vi "Meas Result Generate TWM Digitizer Correction - Process Measurement.vi"(4 "Estimate non-linearity (False)":bool, 5 "digitizer type":T1=enum."HP3458A", 6 "use aperture correction (true)":bool=TRUE, 7 "table ref":refnum<vi>, 8 "error in":errorcluster, 9 "use time shift (true)":bool=TRUE, 10 "Mode":T3, 11 "meas":T4={"swp cfg"={"N"=0, "R"=0, "f list"=[], "smpl delay"=0.0, "set delay"=0.0, "set delay np"=0.0, "meas root"=path "", "meas name"="", "meas a-index"=FALSE, "rnd sweep"=FALSE, "mode"=enum."Frequency", "swp mode"=enum."Linear", "avg"=0, "subrec"=0, "multi-freq"=FALSE, "selfcal"=FALSE, "selfcal period [h]"=0.0}, "bridge"={"type"=enum."TWM client", "TWM"={"pipe name"="", "parameters"=[], "handle"=0, "fixed aper [s]"=0.0, "f-list [Hz]"=[], "discrete f-list"=FALSE, "unc mode"=enum."None", "unc mcc"=0, "unc first"=FALSE, "alg id"=enum."TWM-LowZ - Low Z measurement"}, "last f"=0.0, "bias comp"={"bias type"=enum."dummy", "VISA"="", "Enable"=FALSE, "channel qu"=[], "channel Uinit"=[]}, "sim mode"=enum."Generic RLC network", "channel idns"=[], "sim phases"=1}, "src"={"type"=enum."Tektronix AFG3101C", "afg"={"VISA"="", "const"=0.0, "gen DC"=FALSE, "ext ref"=FALSE}, "cDAQ dds"={"device"="", "channels"=[], "mclk source"="", "mclk [Hz]"=0.0, "fs [Hz]"=0.0, "block [s]"=0.0, "buf [s]"=0.0, "task"="", "cmd queue"=refnum, "proc ref"=refnum, "smpl clock out"="/cDAQ3/PFI0", "export smpl clock"=FALSE, "DC ofs [V]"=[], "timebase source"="", "timebase mode"=enum."Local", "dither"=enum."Disabled", "dither level"=0.0, "phase [rad]"=[]}, "gain [V/A]"=1.0, "F5xxx session"={"VISA"="", "mode"=enum."AC voltage", "Earth on"=FALSE, "Ext ref lock"=FALSE}}, "results"=refnum, "dvm"={"type"=enum."Disabled", "F5790"={"VISA"="", "Input"=enum."input 1", "Digital filter restart"=enum."medium", "hi resolution"=enum."off", "Digital filter mode"=enum."off", "ext guard"=FALSE}}, "thermo"={"type"=enum."COMET Tx5xx (ethernet)", "comment"="", "tag"="", "refresh"=5.0, "IP"="", "port"=502, "VISA"="", "last readout"=timestamp(0 s since 1904-01-01), "TCP ref"=refnum, "VISA sess"="", "idn"="", "press"=0.0, "RH"=0.0, "temp"=0.0, "pres cor"=[], "RH cor"=[], "temp cor"=[], "try left"=0, "failed"=FALSE, "RTD set"=[], "RTD inv"=[], "range"=0.0, "net mode"=enum."MODBUS", "try fail"=enum."Stop trying - return NaN", "timeout [s]"=0.0, "max retries"=0, "sim t [deg]"=0.0}} {"thermo"."RTD inv" format="%.1f"; "thermo"."RTD set" format="%.1f"; "thermo"."temp cor" format="%.1f"; "thermo"."RH cor" format="%.1f"; "thermo"."pres cor" format="%.1f"; "thermo"."refresh" min=0.1 max=1000.0 format="%.2f"; "src"."cDAQ dds"."channels" min=0 step=1; "bridge"."TWM"."f-list [Hz]" format="%#_6p"; "swp cfg"."f list"."bias" format="%#_3p"; "swp cfg"."f list"."level" format="%#_3p"; "swp cfg"."f list"."fs [Hz]" format="%#_5p"; "swp cfg"."f list"."time [s]" format="%#_3p"; "swp cfg"."f list"."f/fs" format="%#_3p"; "swp cfg"."f list"."periods" format="%#_3f"; "swp cfg"."f list"."f [Hz]" format="%#_5p"}) -> (0 "error out":errorcluster, 3 "correction data":T2)   [LabVIEW 2020]
doc: "Generates simple TWM digitizer correction from measured data."
uses:
  meas session.ctl
  Meas Sweep Config.ctl
  Meas Freq Info.ctl
  meas_swp_mode.ctl
  meas_sweep_flist_mode.ctl
  bridge/Bridge Session.ctl
  bridge/Bridge Type.ctl
  drivers/TWM client/TWM Session.ctl
  drivers/TWM client/TWM parameters.ctl
  drivers/TWM client/Meas Proc QWTB Uncertainty Mode.ctl
  bridge/Bridge Algorithm.ctl
  bridge/Bridge Bias Session.ctl
  bridge/Bridge Bias Type.ctl
  bridge/Bridge Sim Mode.ctl
  source/Source Session.ctl
  source/Source Type.ctl
  drivers/AFG3101C/AFG3101C Session.ctl
  drivers/cDAQ DDS/cDAQ DDS Session.ctl
  drivers/cDAQ DDS/cDAQ DDS Setup.ctl
  drivers/cDAQ DDS/cDAQ DDS Timebase Mode.ctl
  drivers/cDAQ DDS/cDAQ DDS Dither.ctl
  drivers/Fluke 5XXX/top_lev/F5xxx_session.ctl
  drivers/Fluke 5XXX/top_lev/F5xxx_output_mode.ctl
  results/Meas Results Ref.ctl
  results/Meas Results.ctl
  bridge/Bridge Frequency Readings Data.ctl
  drivers/TWM client/Meas Proc QWTB Spectrum Data.ctl
  drivers/TWM client/TWM Phase Info.ctl
  dvm/dvm session.ctl
  dvm/dvm type.ctl
  drivers/Fluke 5790A/top_level/F5790 session.ctl
  thermo/thermo.ctl
  thermo/thermo_types.ctl
  thermo/Thermometer Fail Action.ctl
  results/Meas Results Correction Structuring Mode.ctl
  Meas Results TWM Digitizer Correction Data.ctl
  Meas Results TWM Correction Digitizer Type.ctl
  results/Meas Results Sweep Data Uncertainty Mode.ctl
  results/Impedance Equivalent Circuit.ctl
panel:
  out "time shifts [s]":dbl[][](array[numeric]) format="%#_6p"
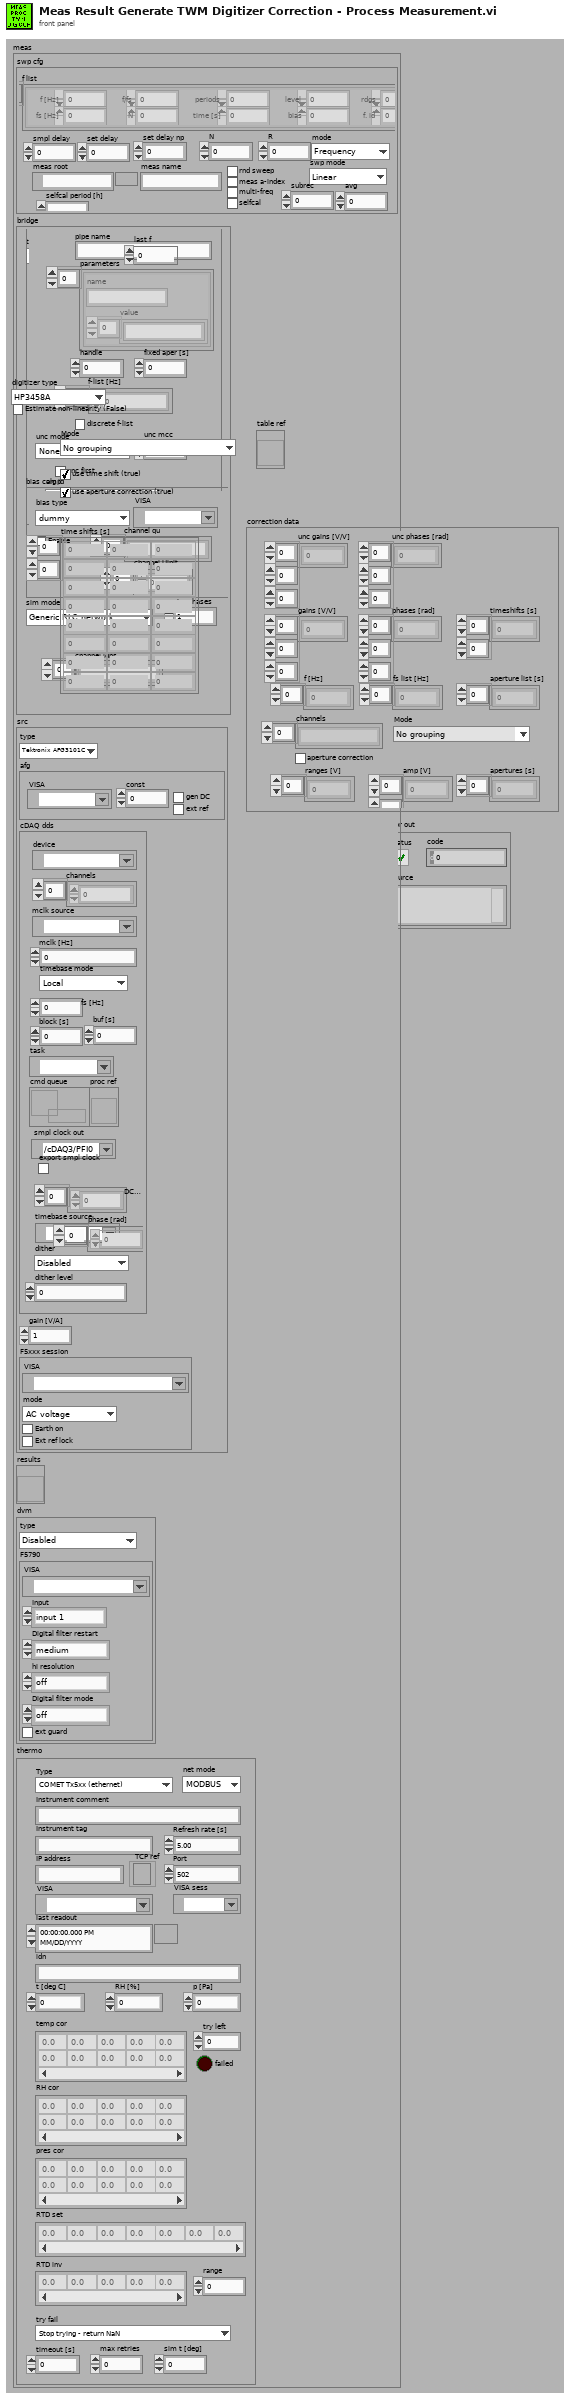
[diagram p1: front panel]
types:
  T1 = typedef "Meas Results TWM Correction Digitizer Type.ctl" = enum16{"Unknown", "HP3458A", "NI9238"}
  T2 = typedef "Meas Results TWM Digitizer Correction Data.ctl" = cluster{"gains [V/V]":dbl[][][], "phases [rad]":dbl[][][], "timeshifts [s]":dbl[][], "f [Hz]":dbl[], "fs list [Hz]":dbl[], "aperture list [s]":dbl[], "channels":string[], "Mode":T3, "aperture correction":bool, "ranges [V]":dbl[], "amp [V]":dbl[][], "apertures [s]":dbl[], "unc gains [V/V]":dbl[][][], "unc phases [rad]":dbl[][][]}
  T3 = typedef "Meas Results Correction Structuring Mode.ctl" = enum16{"No grouping", "Group by apertures (3458A)", "Group by fs (generic digitizer)"}
  T4 = typedef "meas session.ctl" = cluster{"swp cfg":T5, "bridge":T9, "src":T18, "results":T26, "dvm":T27, "thermo":T30}
  T5 = typedef "Meas Sweep Config.ctl" = cluster{"N":i32, "R":i32, "f list":T6[], "smpl delay":dbl, "set delay":dbl, "set delay np":dbl, "meas root":path, "meas name":string, "meas a-index":bool, "rnd sweep":bool, "mode":T7, "swp mode":T8, "avg":i32, "subrec":i32, "multi-freq":bool, "selfcal":bool, "selfcal period [h]":dbl}
  T6 = typedef "Meas Freq Info.ctl" = cluster{"f [Hz]":dbl, "periods":dbl, "f/fs":dbl, "time [s]":dbl, "fs [Hz]":dbl, "N":i32, "level":dbl, "bias":dbl, "rdgs":i32, "f. id":i32}
  T7 = typedef "meas_swp_mode.ctl" = enum16{"Frequency", "Level", "Bias"}
  T8 = typedef "meas_sweep_flist_mode.ctl" = enum16{"Linear", "Log10"}
  T9 = typedef "Bridge Session.ctl" = cluster{"type":T10, "TWM":T11, "last f":dbl, "bias comp":T15, "sim mode":T17, "channel idns":string[], "sim phases":i32}
  T10 = typedef "Bridge Type.ctl" = enum16{"TWM client", "dummy"}
  T11 = typedef "TWM Session.ctl" = cluster{"pipe name":string, "parameters":T12[], "handle":i32, "fixed aper [s]":dbl, "f-list [Hz]":dbl[], "discrete f-list":bool, "unc mode":T13, "unc mcc":i32, "unc first":bool, "alg id":T14}
  T12 = typedef "TWM parameters.ctl" = cluster{"name":string, "value":string[]}
  T13 = typedef "Meas Proc QWTB Uncertainty Mode.ctl" = enum16{"None", "GUF", "Monte Carlo"}
  T14 = typedef "Bridge Algorithm.ctl" = enum16{"TWM-LowZ - Low Z measurement", "TWM-InpZ - Digitizer input Z measurement", "TWM-TIAZ - High Z using TIA"}
  T15 = typedef "Bridge Bias Session.ctl" = cluster{"bias type":T16, "VISA":refnum<visa-resource-name>, "Enable":bool, "channel qu":string[], "channel Uinit":dbl[]}
  T16 = typedef "Bridge Bias Type.ctl" = enum16{"dummy", "CMI LiBbias V1.0"}
  T17 = typedef "Bridge Sim Mode.ctl" = enum16{"Generic RLC network", "Interchannel transfer", "Input impedance"}
  T18 = typedef "Source Session.ctl" = cluster{"type":T19, "afg":T20, "cDAQ dds":T21, "gain [V/A]":dbl, "F5xxx session":T24}
  T19 = typedef "Source Type.ctl" = enum16{"Tektronix AFG3101C", "cDAQ DAC", "Fluke 5xxx", "Agilent 33120A", "dummy"}
  T20 = typedef "AFG3101C Session.ctl" = cluster{"VISA":refnum<visa-resource-name>, "const":dbl, "gen DC":bool, "ext ref":bool}
  T21 = typedef "cDAQ DDS Session.ctl" = cluster{"device":tag, "channels":i32[], "mclk source":tag, "mclk [Hz]":dbl, "fs [Hz]":dbl, "block [s]":dbl, "buf [s]":dbl, "task":refnum<k21>, "cmd queue":refnum<queue>, "proc ref":refnum<vi>, "smpl clock out":tag, "export smpl clock":bool, "DC ofs [V]":dbl[], "timebase source":tag, "timebase mode":T22, "dither":T23, "dither level":dbl, "phase [rad]":dbl[]}
  T22 = typedef "cDAQ DDS Timebase Mode.ctl" = enum16{"Local", "Take from ADC (e.g. NI 9238)", "Other source"}
  T23 = typedef "cDAQ DDS Dither.ctl" = enum16{"Disabled", "Gaussian"}
  T24 = typedef "F5xxx_session.ctl" = cluster{"VISA":refnum<visa-resource-name>, "mode":T25, "Earth on":bool, "Ext ref lock":bool}
  T25 = typedef "F5xxx_output_mode.ctl" = enum16{"AC voltage", "AC current"}
  T26 = typedef "Meas Results Ref.ctl" = refnum<vi>
  T27 = typedef "dvm session.ctl" = cluster{"type":T28, "F5790":T29}
  T28 = typedef "dvm type.ctl" = enum16{"Disabled", "Simulated", "Fluke 5790A"}
  T29 = typedef "F5790 session.ctl" = cluster{"VISA":refnum<visa-resource-name>, "Input":enum16{"input 1", "input 2", "wide-band"}, "Digital filter restart":enum16{"medium", "fine", "coarse"}, "hi resolution":enum16{"off", "on"}, "Digital filter mode":enum16{"off", "fast", "medium", "slow"}, "ext guard":bool}
  T30 = typedef "thermo.ctl" = cluster{"type":T31, "comment":string, "tag":string, "refresh":dbl, "IP":string, "port":u16, "VISA":refnum<visa-resource-name>, "last readout":timestamp, "TCP ref":refnum<k5>, "VISA sess":refnum<visa-resource-name>, "idn":string, "press":dbl, "RH":dbl, "temp":dbl, "pres cor":dbl[][], "RH cor":dbl[][], "temp cor":dbl[][], "try left":i32, "failed":bool, "RTD set":dbl[], "RTD inv":dbl[], "range":dbl, "net mode":enum16{"MODBUS", "HTTP"}, "try fail":T32, "timeout [s]":dbl, "max retries":i32, "sim t [deg]":dbl}
  T31 = typedef "thermo_types.ctl" = enum16{"Disabled", "Simulated", "COMET Tx5xx (ethernet)", "Keithley 2002 (GPIB) + RTD", "Agilent 344xx (GPIB) + RTD"}
  T32 = typedef "Thermometer Fail Action.ctl" = enum16{"Stop trying - keep last value", "Stop trying - return NaN", "Generate error - stop sweep"}
  T33 = typedef "Meas Results Sweep Data Uncertainty Mode.ctl" = enum16{"ua(y)", "ua(y) (p=95%)", "uc(y) (p=95%)"}
  T34 = typedef "Meas Results.ctl" = cluster{"freqs":T35[][], "locked":bool, "last fid":i32, "modified":bool, "mjr name":string, "mnr name":string, "last spectra":T36[][], "saved?":bool, "TWM phase":T37[], "time start":timestamp, "time stop":timestamp, "equ cct":string}
  T35 = typedef "Bridge Frequency Readings Data.ctl" = cluster{"Udut":dbl[], "Iref":dbl[], "Udc":dbl[], "Idc":dbl[], "mjr":dbl[], "mnr":dbl[], "mjr_sh":dbl[], "mnr_sh":dbl[], "u(mjr)":dbl[], "u(mnr)":dbl[], "ua2(mjr)":dbl[], "ua2(mnr)":dbl[], "n":i32, "f [Hz]":dbl, "fs [Hz]":dbl, "aperture [s]":dbl, "Udvm":dbl[], "u(Udvm) [V]":dbl, "t_dut [degC]":dbl[], "RH_dut [%]":dbl[], "p_dut [Pa]":dbl[]}
  T36 = typedef "Meas Proc QWTB Spectrum Data.ctl" = cluster{"x":sgl[], "y":sgl[], "label":string}
  T37 = typedef "TWM Phase Info.ctl" = cluster{"ref chn id (I)":string, "dut chn id (U)":string, "ref chn range [V]":dbl, "dut chn range [V]":dbl, "aperture [s]":dbl, "fs [Hz]":dbl, "ref chn transducer (I)":string, "dut chn transducer (U)":string}
  T38 = typedef "Impedance Equivalent Circuit.ctl" = enum16{"Keep original", "Rs-Xs", "Gp-Bp", "Z-phid", "Z-phir", "Y-phid", "Y-phir", "Cp-D", "Cp-Q", "Cp-Rp", "Cp-Gp", "Cs-D", "Cs-Q", "Cs-Rs", "Ls-Rs", "Ls-Q", "Rs-Tau"}
  T39 = typedef "Meas Results Sweep Data.ctl" = cluster{"Udut":dbl[], "Iref":dbl[], "Udc":dbl[], "Idc":dbl[], "mjr":dbl[], "mnr":dbl[], "mjr_sh":dbl[], "mnr_sh":dbl[], "f [Hz]":dbl[], "n [-]":i32[], "fs [Hz]":dbl[], "aperture [s]":dbl[], "Udvm":dbl[], "t_dut [degC]":dbl[], "RH_dut [%]":dbl[], "p_dut [Pa]":dbl[]}
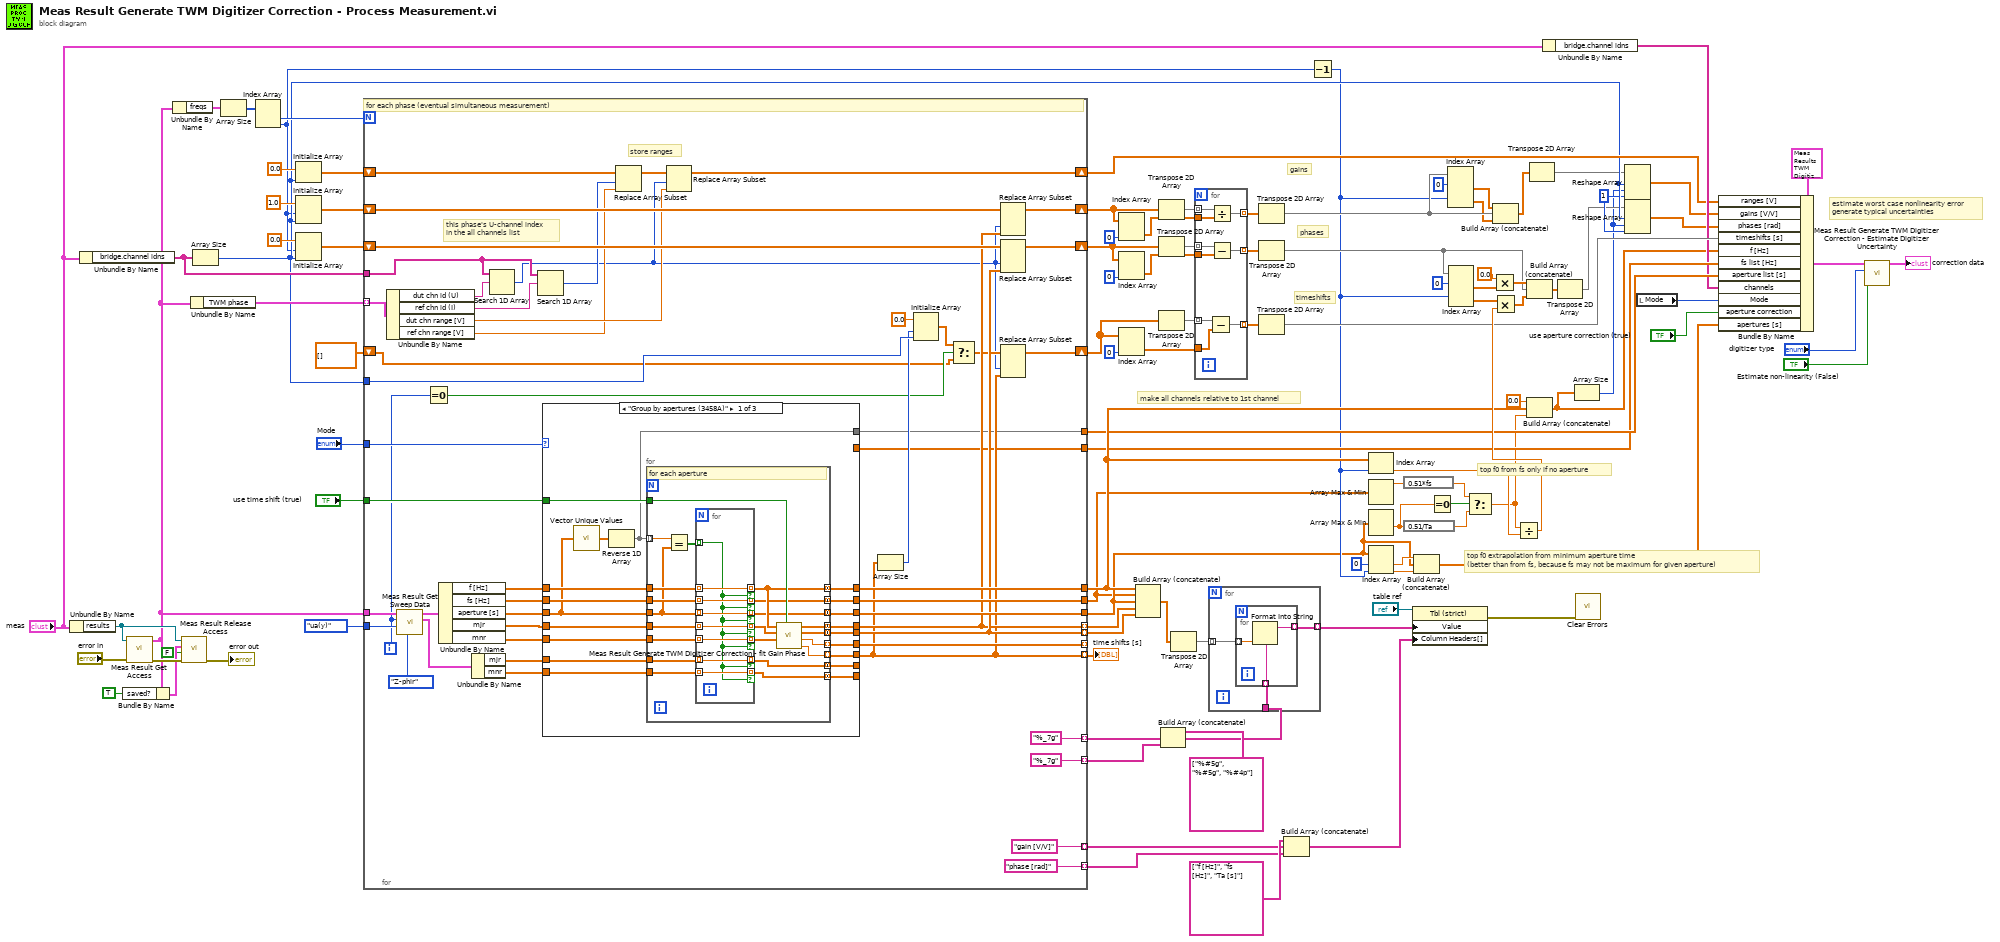
[diagram p0: block diagram]
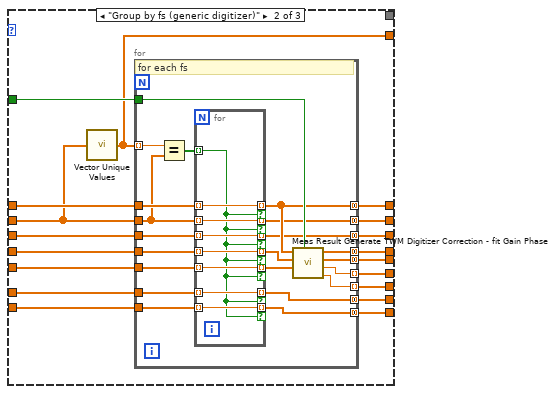
[diagram p2: hidden frame]
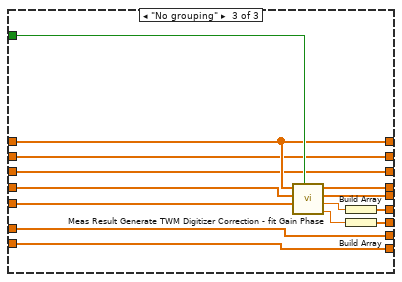
[diagram p3: hidden frame]
diagram:
  w17 = 1 ("dimension size")
  # "top f0 from fs only if no aperture"
  # "top f0 extrapolation from minimum aperture time\n(better than from fs, because fs may not be maximum for given aperture)"
  # "estimate worst case nonlinearity error\ngenerate typical uncertainties"
  # "timeshifts"
  # "phases"
  # "gains"
  # "make all channels relative to 1st channel"
  n1 = Unbundle By Name("meas") -> ("results"=w99:T26)
  n2 = Unbundle By Name("meas") -> ("bridge.channel idns"=w82:string[])
  n3 = call "Meas Result Get Access.vi"("error in"="error in", "results ref"=w99) -> ("error out"=w102:errorcluster, "results data"=w81:T34)  [unwired: 8 in]
  n4 = Bundle By Name(cluster=w81, "saved?"=TRUE) -> (w100:T34)
  n5 = Unbundle By Name(w81) -> ("freqs"=w105:T35[][])
  n6 = call "Meas Result Release Access.vi"("error in"=w102, "Release only (True)"=FALSE, "results data in"=w100, "results ref"=w99) -> ("error out"=→"error out":errorcluster)  [unwired: 7 in]
  n7 = Unbundle By Name(w81) -> ("TWM phase"=w80:T37[])
  n8 = Array Size(array=w82) -> (size(s)=w20:i32)
  n9 = Array Size(array=w105) -> (size(s)=w104:i32[])
  n10 = Index Array(array=w104) -> (element #1=w103:i32, element #2=w18:i32)  [unwired: 2 in]
  n11 = Initialize Array(0.0 ("element"), w20) -> (w30:dbl[])
  n12 = Initialize Array(1.0 ("element"), w18, w20) -> (w78:dbl[][])
  n13 = Initialize Array(0.0 ("element"), w18, w20) -> (w83:dbl[][])
  n14 = for {
    N: w103 -> [_]
    tunnel: Meas_Results_Sweep_Data_Uncertainty_Mode."ua(y)" ("uncertainty mode") -> [w156]
    tunnel: w81 -> [w141]
    tunnel: "Mode" -> [w155]
    tunnel: "use time shift (true)" -> [w150]
    tunnel: [w149] -> w46
    tunnel: [w148] -> w6
    tunnel: [w147] -> w8
    tunnel: [w136] -> w91 mode=indexing
    tunnel: [w142] -> w90 mode=indexing
    tunnel: [w133] -> _ mode=indexing
    tunnel: [w125] -> w85 mode=indexing
    tunnel: ["%_7g"] -> w88 mode=indexing
    tunnel: ["%_7g"] -> w87 mode=indexing
    shift-right: [w143] -> w73
    shift-left: w83 -> [w144]
    tunnel: w82 -> [w115]
    tunnel: w80 -> [w140] mode=indexing
    shift-right: [w138] -> w76
    shift-left: w78 -> [w137]
    shift-right: [w126] -> w67
    shift-left: dbl[][] [] -> [w128]
    tunnel: w20 -> [w134]
    tunnel: [w124] -> w44
    tunnel: [w123] -> w43
    tunnel: ["gain [V/V]"] -> w37 mode=indexing
    tunnel: ["phase [rad]"] -> w36 mode=indexing
    shift-right: [w116] -> w29
    shift-left: w30 -> [w112]
    i -> [w131]
    # "store ranges"
    # "this phase's U-channel index\nin the all channels list"
    # "for each phase (eventual simultaneous measurement)"
    n15 = Unbundle By Name(w140) -> ("dut chn id (U)"=w139:string, "ref chn id (I)"=w114:string, "dut chn range [V]"=w110:dbl, "ref chn range [V]"=w109:dbl)
    n16 = call "Meas Result Get Sweep Data.vi"("equ connection override"=Impedance_Equivalent_Circuit."Z-phir", "uncertainty mode"=w156, "phase index (default: 0)"=w131, "result"=w141) -> ("unc(data)"=w119:T39, "data"=w157:T39)  [unwired: 5 in, 1 out]
    n17 = Equal To 0?(x=w131) -> (x = 0?=w130:bool)
    n18 = Unbundle By Name(w157) -> ("f [Hz]"=w154:dbl[], "fs [Hz]"=w153:dbl[], "aperture [s]"=w152:dbl[], "mjr"=w120:dbl[], "mnr"=w151:dbl[])
    n19 = Unbundle By Name(w119) -> ("mjr"=w118:dbl[], "mnr"=w117:dbl[])
    n20 = Search 1D Array(1D array=w115, element=w139) -> (index of element=w108:i32)  [unwired: 1 in]
    n21 = Search 1D Array(1D array=w115, element=w114) -> (index of element=w111:i32)  [unwired: 1 in]
    n22 = case shown="\"Group by apertures (3458A)\"" w155 {
      tunnel: w154 -> [w176 w223 w263]
      tunnel: w153 -> [w175 w218 w256]
      tunnel: w152 -> [w172 w220 w255]
      tunnel: w120 -> [w174 w222 w266]
      tunnel: w151 -> [w173 w221 w265]
      tunnel: w150 -> [w170 w219 w264]
      tunnel: [w169 w217 w263] -> w149
      tunnel: [w168 w216 w256] -> w148
      tunnel: [w167 w215 w255] -> w147
      tunnel: [w166 w214 w262] -> w136
      tunnel: [w165 w213 w261] -> w142
      tunnel: [w164 w212 w257] -> w133
      tunnel: [w163 w211 w258] -> w125
      tunnel: [w162 _ _] -> w124
      tunnel: [_ w210 _] -> w123
      tunnel: w118 -> [w161 w209 w253]
      tunnel: w117 -> [w160 w208 w254]
      tunnel: [w159 w207 w253] -> _
      tunnel: [w158 w206 w254] -> _
      frame "Group by apertures (3458A)" {
        n23 = call "Vector Unique Values.vi"("array in"=w172) -> ("uniques out"=w171:dbl[])
        n24 = Reverse 1D Array(array=w171) -> (reversed array=w162:dbl[])
        n25 = for {
          tunnel: w176 -> [w195]
          tunnel: w175 -> [w194]
          tunnel: w172 -> [w193]
          tunnel: w174 -> [w192]
          tunnel: w173 -> [w191]
          tunnel: w162 -> [w197] mode=indexing
          tunnel: w170 -> [w188]
          tunnel: [w187] -> w169 mode=concatenating
          tunnel: [w186] -> w168 mode=concatenating
          tunnel: [w185] -> w167 mode=concatenating
          tunnel: [w184] -> w166 mode=concatenating
          tunnel: [w183] -> w165 mode=concatenating
          tunnel: [w182] -> w164 mode=indexing
          tunnel: [w181] -> w163 mode=indexing
          tunnel: w161 -> [w180]
          tunnel: w160 -> [w179]
          tunnel: [w178] -> w159 mode=concatenating
          tunnel: [w177] -> w158 mode=concatenating
          # "for each aperture"
          n26 = Equal?(x=w197, y=w193) -> (x = y?=w196:bool[])
          n27 = for {
            tunnel: w196 -> [w198] mode=indexing
            tunnel: [w205] -> w187 mode=indexing if=w198
            tunnel: w195 -> [w205] mode=indexing
            tunnel: [w204] -> w186 mode=indexing if=w198
            tunnel: w194 -> [w204] mode=indexing
            tunnel: [w203] -> w185 mode=indexing if=w198
            tunnel: w193 -> [w203] mode=indexing
            tunnel: [w202] -> w190 mode=indexing if=w198
            tunnel: w192 -> [w202] mode=indexing
            tunnel: [w201] -> w189 mode=indexing if=w198
            tunnel: w191 -> [w201] mode=indexing
            tunnel: [w200] -> w178 mode=indexing if=w198
            tunnel: w180 -> [w200] mode=indexing
            tunnel: [w199] -> w177 mode=indexing if=w198
            tunnel: w179 -> [w199] mode=indexing
          }
          n28 = call "Meas Result Generate TWM Digitizer Correction - fit Gain Phase.vi"("use time shift (true)"=w188, "phase [rad]"=w189, "gain [V/V]"=w190, "f [Hz]"=w187) -> ("time shift [s]"=w181:dbl, "DC gain"=w182:dbl, "phase out [rad]"=w183:dbl[], "gain out [V/V]"=w184:dbl[])  [unwired: 4 in]
        }
      }
      frame "Group by fs (generic digitizer)" {
        n29 = call "Vector Unique Values.vi"("array in"=w218) -> ("uniques out"=w210:dbl[])
        n30 = for {
          tunnel: w223 -> [w242]
          tunnel: w218 -> [w228]
          tunnel: w220 -> [w241]
          tunnel: w222 -> [w240]
          tunnel: w221 -> [w239]
          tunnel: w210 -> [w244] mode=indexing
          tunnel: w219 -> [w236]
          tunnel: [w235] -> w217 mode=concatenating
          tunnel: [w234] -> w216 mode=concatenating
          tunnel: [w233] -> w215 mode=concatenating
          tunnel: [w232] -> w214 mode=concatenating
          tunnel: [w231] -> w213 mode=concatenating
          tunnel: [w230] -> w212 mode=indexing
          tunnel: [w229] -> w211 mode=indexing
          tunnel: w209 -> [w227]
          tunnel: w208 -> [w226]
          tunnel: [w225] -> w207 mode=concatenating
          tunnel: [w224] -> w206 mode=concatenating
          # "for each fs"
          n31 = Equal?(x=w244, y=w228) -> (x = y?=w243:bool[])
          n32 = for {
            tunnel: w243 -> [w245] mode=indexing
            tunnel: [w252] -> w235 mode=indexing if=w245
            tunnel: w242 -> [w252] mode=indexing
            tunnel: [w251] -> w234 mode=indexing if=w245
            tunnel: w228 -> [w251] mode=indexing
            tunnel: [w250] -> w233 mode=indexing if=w245
            tunnel: w241 -> [w250] mode=indexing
            tunnel: [w249] -> w238 mode=indexing if=w245
            tunnel: w240 -> [w249] mode=indexing
            tunnel: [w248] -> w237 mode=indexing if=w245
            tunnel: w239 -> [w248] mode=indexing
            tunnel: [w247] -> w225 mode=indexing if=w245
            tunnel: w227 -> [w247] mode=indexing
            tunnel: w226 -> [w246] mode=indexing
            tunnel: [w246] -> w224 mode=indexing if=w245
          }
          n33 = call "Meas Result Generate TWM Digitizer Correction - fit Gain Phase.vi"("use time shift (true)"=w236, "phase [rad]"=w237, "gain [V/V]"=w238, "f [Hz]"=w235) -> ("time shift [s]"=w229:dbl, "DC gain"=w230:dbl, "phase out [rad]"=w231:dbl[], "gain out [V/V]"=w232:dbl[])  [unwired: 4 in]
        }
      }
      frame "No grouping" {
        n34 = call "Meas Result Generate TWM Digitizer Correction - fit Gain Phase.vi"("use time shift (true)"=w264, "phase [rad]"=w265, "gain [V/V]"=w266, "f [Hz]"=w263) -> ("time shift [s]"=w259:dbl, "DC gain"=w260:dbl, "phase out [rad]"=w261:dbl[], "gain out [V/V]"=w262:dbl[])  [unwired: 4 in]
        n35 = Build Array(w260) -> (w257:dbl[])
        n36 = Build Array(w259) -> (w258:dbl[])
      }
    }
    n37 = Replace Array Subset(array=w112, new element=w109, index=w111) -> (w113:dbl[])
    n38 = Replace Array Subset(array=w113, new element=w110, index=w108) -> (w116:dbl[])
    n39 = Array Size(array=w125) -> (size(s)=w132:i32)
    n40 = Initialize Array(0.0 ("element"), w132, w134) -> (w129:dbl[][])
    n41 = Select(t=w129, s=w130, f=w128) -> (s? t:f=w127:dbl[][])
    n42 = Replace Array Subset(array=w137, new element=w136, index (col)=w108) -> (w138:dbl[][])  [unwired: 1 in]
    n43 = Replace Array Subset(array=w144, new element=w142, index (col)=w108) -> (w143:dbl[][])  [unwired: 1 in]
    n44 = Replace Array Subset(array=w127, new element=w125, index (col)=w108) -> (w126:dbl[][])  [unwired: 1 in]
  }
  "time shifts [s]" <- w85
  n45 = Index Array(array=w76, index (col)=0 ("disabled index (col)")) -> (element=w75:dbl[])  [unwired: 1 in]
  n46 = Index Array(array=w73, index (col)=0 ("disabled index (col)")) -> (element=w72:dbl[])  [unwired: 1 in]
  n47 = Index Array(array=w67, index (col)=0 ("disabled index (col)")) -> (element=w68:dbl[])  [unwired: 1 in]
  n48 = Build Array (concatenate)(w46, w6, w8, w91, w90) -> (w94:dbl[][])
  n49 = Transpose 2D Array(2D array=w76) -> (transposed array=w66:dbl[][])
  n50 = Transpose 2D Array(2D array=w73) -> (transposed array=w65:dbl[][])
  n51 = Transpose 2D Array(2D array=w67) -> (transposed array=w64:dbl[][])
  n52 = Build Array (concatenate)(string[] ["%#5g", "%#5g", "%#4p"], w88, w87) -> (w86:string[])
  n53 = Transpose 2D Array(2D array=w94) -> (transposed array=w95:dbl[][])
  n54 = for {
    tunnel: w66 -> [w275] mode=indexing
    tunnel: w75 -> [w274]
    tunnel: w65 -> [w273] mode=indexing
    tunnel: w72 -> [w272]
    tunnel: [w271] -> w62 mode=indexing
    tunnel: [w270] -> w71 mode=indexing
    tunnel: w64 -> [w269] mode=indexing
    tunnel: w68 -> [w268]
    tunnel: [w267] -> w63 mode=indexing
    n55 = Subtract(x=w269, y=w268) -> (x-y=w267:dbl[])
    n56 = Divide(x=w275, y=w274) -> (x/y=w271:dbl[])
    n57 = Subtract(x=w273, y=w272) -> (x-y=w270:dbl[])
  }
  n58 = for {
    tunnel: w95 -> [w277] mode=indexing
    tunnel: w86 -> [w278]
    tunnel: [w276] -> w34 mode=indexing
    n59 = for {
      tunnel: w278 -> [w280] mode=indexing
      tunnel: w277 -> [w281] mode=indexing
      tunnel: [w279] -> w276 mode=indexing
      n60 = Format Into String(format string=w280, w281) -> (resulting string=w279:string)  [unwired: 2 in, 1 out]
    }
  }
  n61 = Transpose 2D Array(2D array=w62) -> (transposed array=w58:dbl[][])
  n62 = Transpose 2D Array(2D array=w71) -> (transposed array=w49:dbl[][])
  n63 = Transpose 2D Array(2D array=w63) -> (transposed array=w45:dbl[][])
  n64 = Build Array (concatenate)(string[] ["f [Hz]", "fs [Hz]", "Ta [s]"], w37, w36) -> (w33:string[])
  n65 = Decrement(x=w18) -> (x-1=w19:i32)
  n66 = Index Array(array=w46, index=w19) -> (element=w53:dbl)
  n67 = Array Max & Min(array=w6) -> (max value=w7:dbl)  [unwired: 3 out]
  n68 = Array Max & Min(array=w8) -> (min value=w1:dbl)  [unwired: 3 out]
  n69 = Index Array(array=w8, index #1=0 ("index"), index #2=w19) -> (element #1=w27:dbl, element #2=w26:dbl)
  n70 = expression code="0.51*fs"(w7) -> (w5:dbl)
  n71 = expression code="0.51/Ta"(w1) -> (w4:dbl)
  n72 = property class="Tbl (strict)"(reference="table ref", "Value"=w34, "Column Headers[]"=w33) -> (error out=w32:errorcluster)  [unwired: 1 in, 1 out]
  n73 = Build Array (concatenate)(w27, w8, w26) -> (w25:dbl[])
  n74 = Equal To 0?(x=w1) -> (x = 0?=w2:bool)
  n75 = Index Array(array=w58, index (row) #1=0 ("index (row)"), index (row) #2=w19) -> (element #1=w59:dbl[], element #2=w57:dbl[])  [unwired: 2 in]
  n76 = Index Array(array=w49, index (row) #1=0 ("index (row)"), index (row) #2=w19) -> (element #1=w55:dbl[], element #2=w52:dbl[])  [unwired: 2 in]
  n77 = Select(t=w5, s=w2, f=w4) -> (s? t:f=w3:dbl)
  n78 = Multiply(x=0.0 ("element"), y=w55) -> (x*y=w50:dbl[])
  n79 = Build Array (concatenate)(w59, w58, w57) -> (w24:dbl[][])
  n80 = Divide(x=w3, y=w53) -> (x/y=w51:dbl)
  n81 = Multiply(x=w52, y=w51) -> (x*y=w48:dbl[])
  n82 = Build Array (concatenate)(w50, w49, w48) -> (w21:dbl[][])
  n83 = Build Array (concatenate)(0.0 ("element"), w46, w3) -> (w10:dbl[])
  n84 = Transpose 2D Array(2D array=w24) -> (transposed array=w15:dbl[][])
  n85 = Unbundle By Name("meas") -> ("bridge.channel idns"=w41:string[])
  n86 = Transpose 2D Array(2D array=w21) -> (transposed array=w16:dbl[][])
  n87 = Array Size(array=w10) -> (size(s)=w9:i32)
  n88 = call <vilib>:"Clear Errors.vi"("error in (no error)"=w32) -> ()  [unwired: 5 in, 2 out]
  n89 = Reshape Array(w15, w20, w9, w17) -> (w23:dbl[][][])
  n90 = Reshape Array(w16, w20, w9, w17) -> (w22:dbl[][][])
  n91 = local read "Mode"() -> (w40:T3)
  n92 = Bundle By Name(cluster=T2 {"gains [V/V]"=[], "phases [rad]"=[], "timeshifts [s]"=[], "f [Hz]"=[], "fs list [Hz]"=[], "aperture list [s]"=[], "channels"=[], "Mode"=enum."No grouping", "aperture correction"=FALSE, "ranges [V]"=[], "amp [V]"=[], "apertures [s]"=[], "unc gains [V/V]"=[], "unc phases [rad]"=[]} ("correction data"), "ranges [V]"=w29, "gains [V/V]"=w23, "phases [rad]"=w22, "timeshifts [s]"=w45, "f [Hz]"=w10, "fs list [Hz]"=w43, "aperture list [s]"=w44, "channels"=w41, "Mode"=w40, "aperture correction"="use aperture correction (true)", "apertures [s]"=w25) -> (w14:T2)
  n93 = call "Meas Result Generate TWM Digitizer Correction - Estimate Digitizer Uncertainty.vi"("Estimate non-linearity (False)"="Estimate non-linearity (False)", "digitizer type"="digitizer type", "correction data in"=w14) -> ("correction data out"=→"correction data":T2)  [unwired: 8 in]
